vi "Chronos TDMS Viewer Append New Data.vi"(8 "error in (no error)":errorcluster, 9 "data":dbl[][](array[numeric]), 10 "Ch Names":string[](array[string]), 11 "Plot":T1) -> (0 "error out":errorcluster, 2 "end time":dbl, 3 "Plot out":T1)   [LabVIEW 2021]
uses:
  GUI/Chronos cluster Map Limit Plots.ctl
  typedefs/Chronos cluster Plot Data and Limits.ctl
  cluster CC Channel from TDMS.ctl
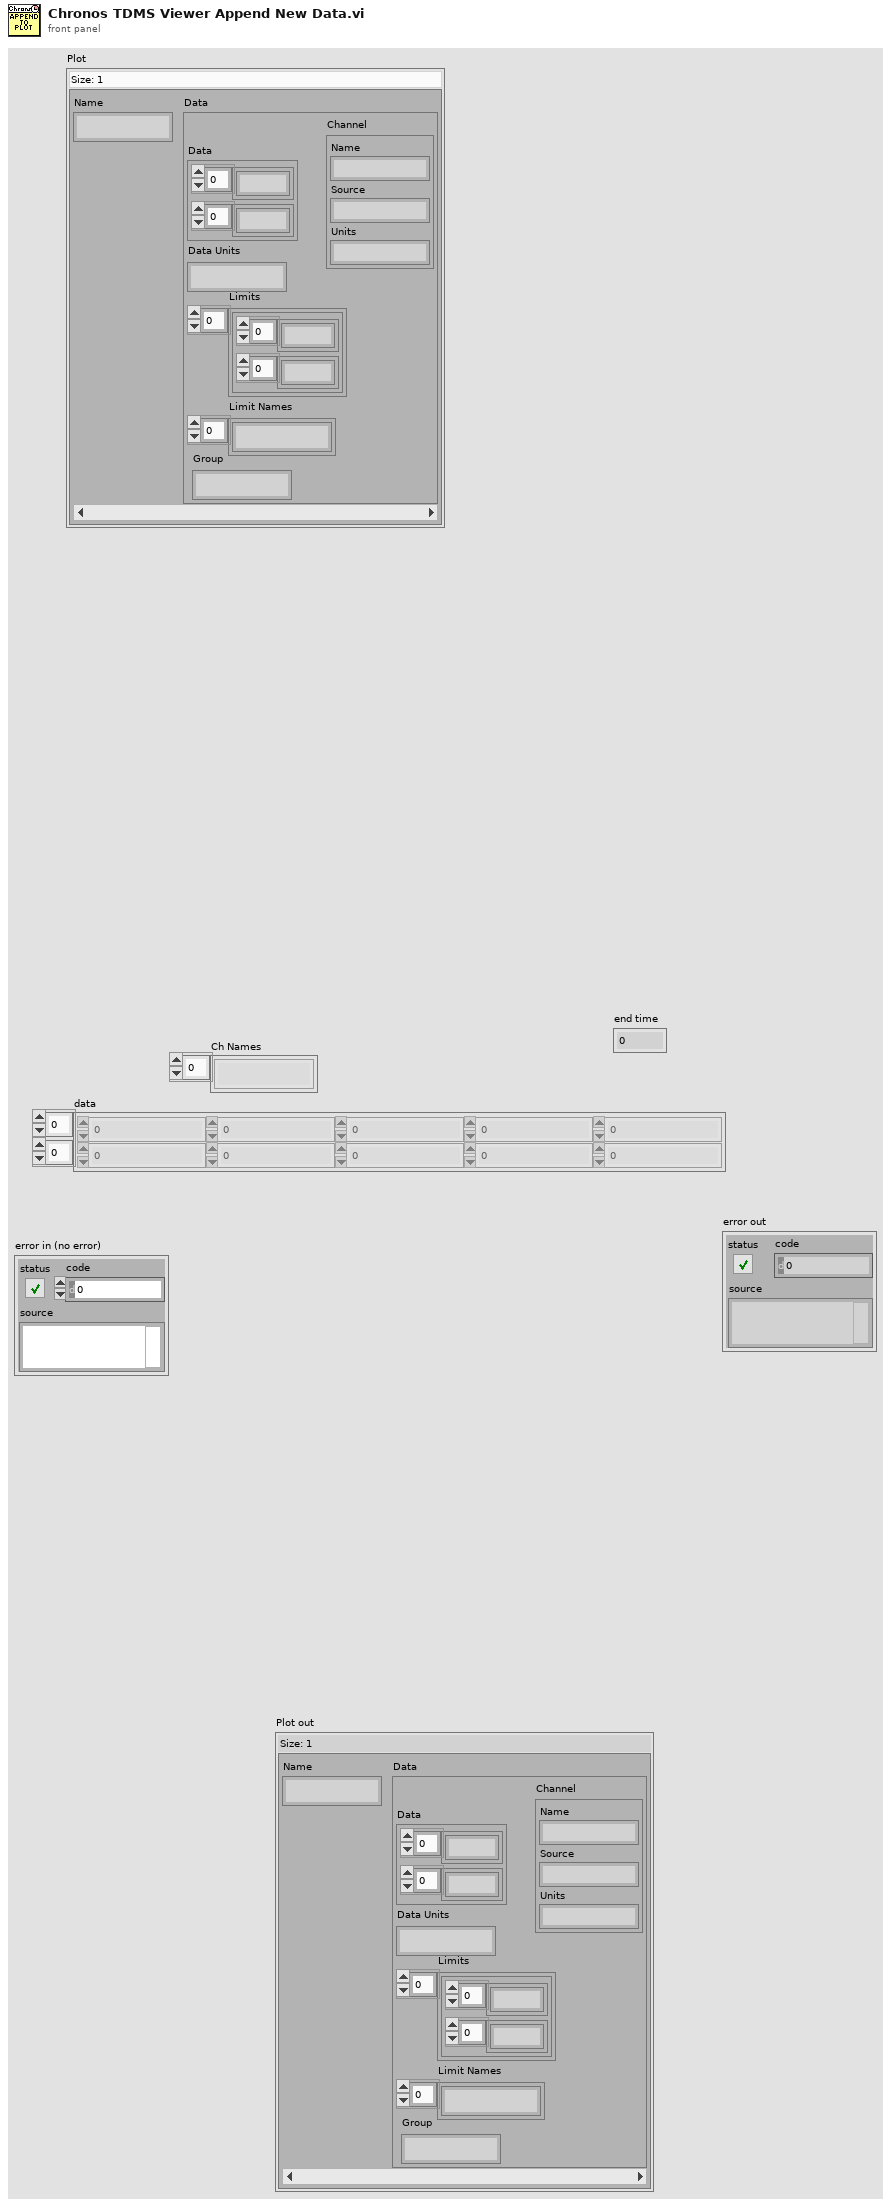
[diagram p1: front panel]
types:
  T1 = typedef "Chronos cluster Map Limit Plots.ctl" = map{string, T2}
  T2 = typedef "Chronos cluster Plot Data and Limits.ctl" = cluster{"Data":cluster{dbl[], dbl[]}, "Data Units":string, "Limits":cluster{dbl[], dbl[]}[], "Limit Names":string[], "Channel":T3, "Group":string}
  T3 = typedef "cluster CC Channel from TDMS.ctl" = cluster{"Name":string, "Source":string, "Units":string}
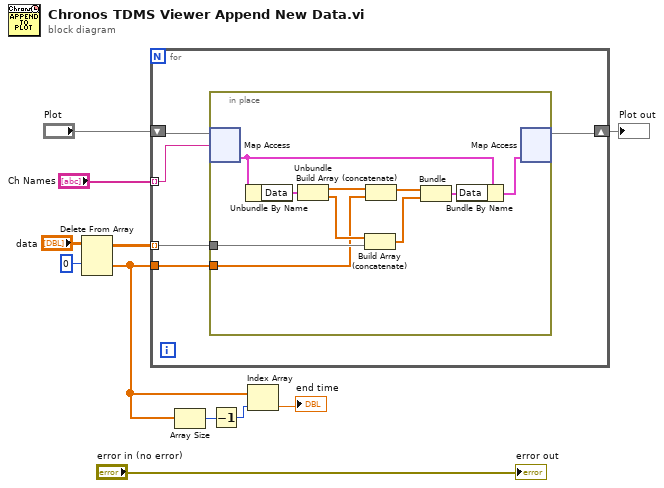
[diagram p0: block diagram]
diagram:
  n1 = Delete From Array(array="data", index (row)=0) -> (deleted portion=w3:dbl[], array with subset deleted=w8:dbl[][])  [unwired: 2 in]
  n2 = for {
    tunnel: "Ch Names" -> [w15] mode=indexing
    shift-right: [w14] -> w2
    shift-left: "Plot" -> [w16]
    tunnel: w8 -> [w13] mode=indexing
    tunnel: w3 -> [w12]
    n3 = in-place {
      in-place-border: w13 -> [w24]
      in-place-border: w12 -> [w22]
      n4 = in-place-map #1(w16, w15) -> (w19:T2)  [unwired: 1 in, 1 out]
      n5 = Unbundle By Name(w19) -> ("Data"=w26:cluster{dbl[], dbl[]})
      n6 = Unbundle(w26) -> (w25:dbl[], w23:dbl[])
      n7 = Build Array (concatenate)(w23, w24) -> (w20:dbl[])
      n8 = Build Array (concatenate)(w25, w22) -> (w21:dbl[])
      n9 = Bundle(w21, w20) -> (w18:cluster{dbl[], dbl[]})  [unwired: 1 in]
      n10 = Bundle By Name(cluster=w19, "Data"=w18) -> (w17:T2)
      n11 = in-place-map #1(w17) -> (w14:T1)  [unwired: 1 in, 2 out]
    }
  }
  "Plot out" <- w2
  n12 = Array Size(array=w3) -> (size(s)=w6:i32)
  n13 = Decrement(x=w6) -> (x-1=w5:i32)
  n14 = Index Array(array=w3, index=w5) -> (element=→"end time":dbl)
  "error out" <- "error in (no error)"
